vi "TDMS File Merge.vi"(0 "serial input channel":string="SI0", 5 "tdms file directory":path, 7 "progress ref":refnum<vi>, 11 "error in":errorcluster) -> (15 "error out":errorcluster)   [LabVIEW 2023, in "GettingStarted_Common_148X_Host.lvlib"]
uses:
  GettingStarted_Common_148X_Host.lvlib
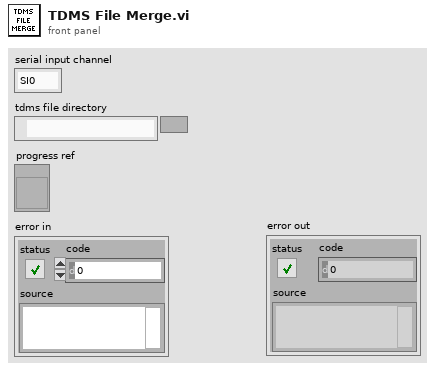
[diagram p1: front panel]
types:
  T1 = enum16{"open", "open or create", "create or replace", "create", "open (read-only)"}
  T2 = enum16{"big-endian, network order", "native, host order", "little-endian"}
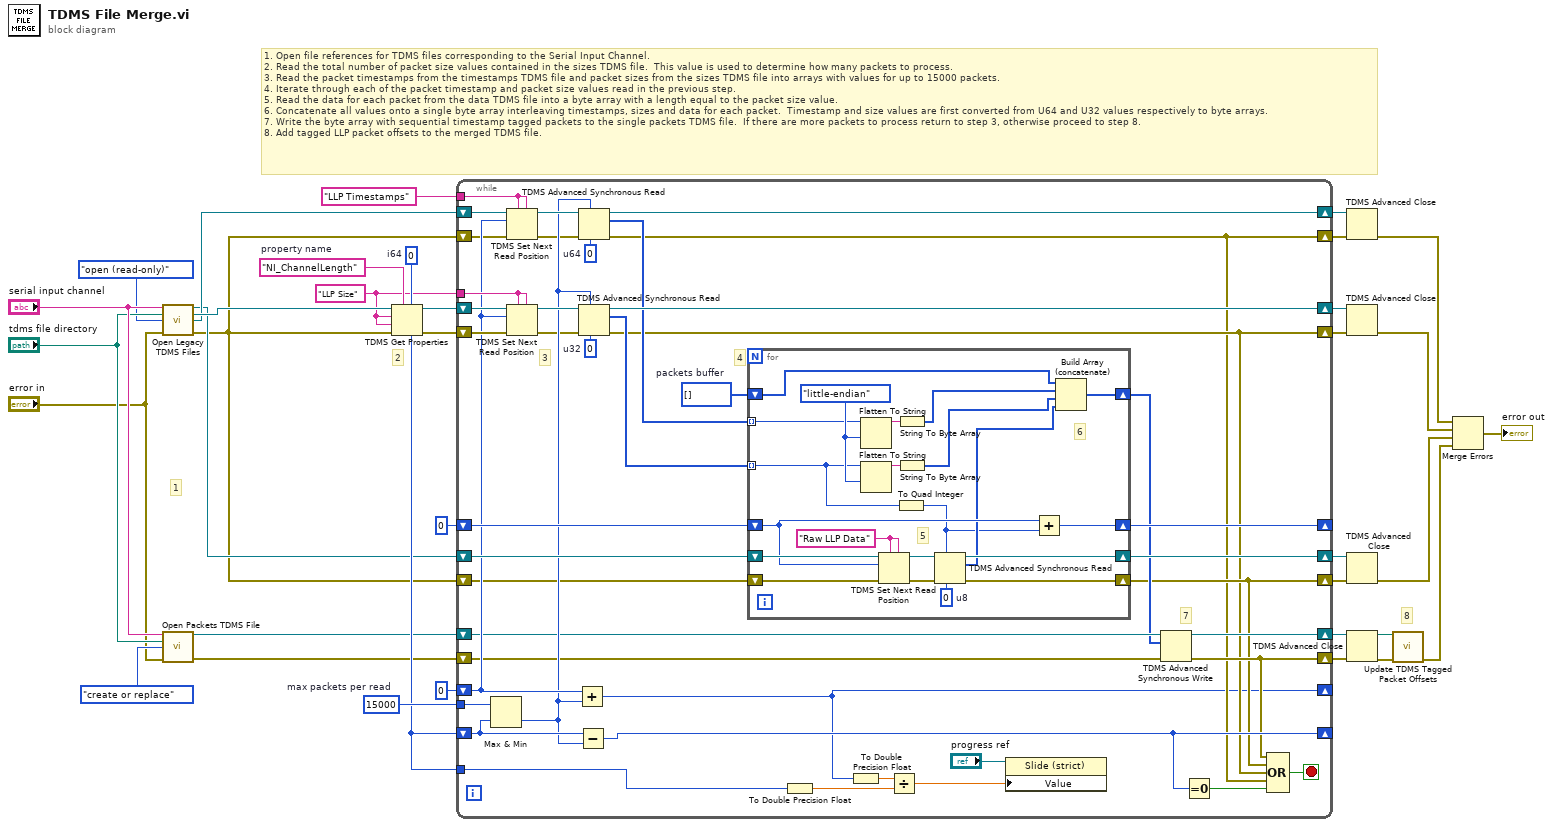
[diagram p0: block diagram]
diagram:
  w33 = i64 15000  # max packets per read
  w16 = "LLP Size" ("channel and group name")
  w35 = i64 0  # i64
  w36 = "NI_ChannelLength"  # property name
  # "2"
  # "8"
  # "1"
  # "1. Open file references for TDMS files corresponding to the Serial Input Channel.\n2. Read the total number of packet size values contained in the sizes TDMS file.  This value is used to determine how many packets to process.\n3. Read the packet timestamps from the timestamps TDMS file and packet sizes from the sizes TDMS file into arrays with values for up to 15000 packets.\n4. Iterate through each of the packet timestamp and packet size values read in the previous step.\n5. Read the data for each packet from the data TDMS file into a byte array with a length equal to the packet size value.\n6. Concatenate all values onto a single byte array interleaving timestamps, sizes and data for each packet.  Timestamp and size values are first converted from U64 and U32 values respectively to byte arrays.\n7. Write the byte array with sequential timestamp tagged packets to the single packets TDMS file.  If there are more packets to process return to step 3, otherwise proceed to step 8.\n8. Add tagged LLP packet offsets to the merged TDMS file."
  n1 = call "Open Legacy TDMS Files.vi"("serial input channel"="serial input channel", "base tdms file path"="tdms file directory", "file operation type"=T1."open (read-only)", "error in (no error)"="error in") -> ("data file ref"=w28:refnum<k34>, "sizes file ref"=w30:refnum<k34>, "timestamp file ref"=w29:refnum<k34>, "error out"=w15:errorcluster)  [unwired: 8 in]
  n2 = call "Open Packets TDMS File.vi"("serial input channel"="serial input channel", "base tdms file path"="tdms file directory", "file operation type"=T1."create or replace", "error in"="error in") -> ("packets file ref"=w23:refnum<k34>, "error out"=w14:errorcluster)  [unwired: 10 in]
  n3 = TDMS Get Properties(5:w35, 7:w36, 8:w15, 9:w16, 10:w16, 11:w30) -> (0:w34:errorcluster, 3:w31:refnum<k34>, 4:w32:i64)  [unwired: 3 out]
  n4 = while {
    shift-right: [w70] -> w17
    shift-left: w29 -> [w73]
    shift-right: [w45] -> w22
    shift-left: w34 -> [w77]
    shift-right: [w53] -> _
    shift-left: w32 -> [w78]
    tunnel: w33 -> [w79]
    tunnel: w32 -> [w39]
    shift-right: [w74] -> w18
    shift-left: w31 -> [w72]
    tunnel: w16 -> [w65]
    shift-right: [w40] -> _
    shift-left: i64 0 -> [w60]
    shift-right: [w63] -> w20
    shift-left: w28 -> [w66]
    shift-right: [w61] -> _
    shift-left: i64 0 ("initial file offset") -> [w64]
    shift-right: [w56] -> w19
    shift-left: w23 -> [w58]
    shift-right: [w46] -> w12
    shift-left: w15 -> [w51]
    shift-right: [w44] -> w13
    shift-left: w15 -> [w52]
    shift-right: [w47] -> w11
    shift-left: w14 -> [w50]
    tunnel: "LLP Timestamps" ("channel and group name") -> [w49]
    stop <- w43 stop-if-true
    w62 = u8[] []  # packets buffer
    w69 = u64 0  # u64
    w75 = u32 0  # u32
    # "4"
    # "7"
    # "3"
    n5 = Max & Min(x=w79, y=w78) -> (min(x,y)=w59:i64)  [unwired: 1 out]
    n6 = TDMS Set Next Read Position(5:w49, 7:w49, 8:w52, 10:w60, 11:w73) -> (0:w54:errorcluster, 3:w71:refnum<k34>)  [unwired: 1 in]
    n7 = TDMS Set Next Read Position(5:w65, 7:w65, 8:w77, 10:w60, 11:w72) -> (0:w55:errorcluster, 3:w76:refnum<k34>)  [unwired: 1 in]
    n8 = Add(x=w60, y=w59) -> (x+y=w40:i64)
    n9 = Subtract(x=w78, y=w59) -> (x-y=w53:i64)
    n10 = TDMS Advanced Synchronous Read(6:w69, 7:w59, 8:w54, 11:w71) -> (0:w44:errorcluster, 2:w67:u64[], 3:w70:refnum<k34>)  [unwired: 1 out]
    n11 = TDMS Advanced Synchronous Read(6:w75, 7:w59, 8:w55, 11:w76) -> (0:w45:errorcluster, 2:w68:u32[], 3:w74:refnum<k34>)  [unwired: 1 out]
    n12 = for {
      tunnel: w68 -> [w81] mode=indexing
      tunnel: w67 -> [w82] mode=indexing
      shift-right: [w93] -> w61
      shift-left: w64 -> [w94]
      shift-right: [w98] -> w46
      shift-left: w51 -> [w88]
      shift-right: [w96] -> w63
      shift-left: w66 -> [w100]
      shift-right: [w90] -> w57
      shift-left: w62 -> [w91]
      w83 = T2."little-endian" ("byte order (0:big-endian, network order)")
      w89 = "Raw LLP Data" ("channel and group name")
      w95 = u8 0  # u8
      # "6"
      # "5"
      n13 = Flatten To String(anything=w82, byte order (0:big-endian, network order)=w83) -> (data string=w85:string)  [unwired: 2 in, 2 out]
      n14 = Flatten To String(anything=w81, byte order (0:big-endian, network order)=w83) -> (data string=w87:string)  [unwired: 2 in, 2 out]
      n15 = TDMS Set Next Read Position(5:w89, 7:w89, 8:w88, 10:w94, 11:w100) -> (0:w99:errorcluster, 3:w97:refnum<k34>)  [unwired: 1 in]
      n16 = To Quad Integer(1:w81) -> (0:w80:i64)
      n17 = String To Byte Array(string=w85) -> (unsigned byte array=w84:u8[])
      n18 = String To Byte Array(string=w87) -> (unsigned byte array=w86:u8[])
      n19 = TDMS Advanced Synchronous Read(6:w95, 7:w80, 8:w99, 11:w97) -> (0:w98:errorcluster, 2:w92:u8[], 3:w96:refnum<k34>)  [unwired: 1 out]
      n20 = Add(x=w94, y=w80) -> (x+y=w93:i64)
      n21 = Build Array (concatenate)(w91, w84, w86, w92) -> (w90:u8[])
    }
    n22 = To Double Precision Float(number=w39) -> (double precision float=w41:dbl)
    n23 = To Double Precision Float(number=w40) -> (double precision float=w42:dbl)
    n24 = Divide(x=w42, y=w41) -> (x/y=w37:dbl)
    n25 = property class="Slide (strict)"(reference="progress ref", "Value"=w37) -> ()  [unwired: 1 in, 2 out]
    n26 = TDMS Advanced Synchronous Write(8:w50, 10:w57, 11:w58) -> (0:w47:errorcluster, 3:w56:refnum<k34>)
    n27 = Equal To 0?(x=w53) -> (x = 0?=w48:bool)
    n28 = Compound Arithmetic op=OR(w47, w46, w45, w44, w48) -> (w43:bool)
  }
  n29 = TDMS Advanced Close(8:w13, 11:w17) -> (0:w8:errorcluster)  [unwired: 2 in, 1 out]
  n30 = TDMS Advanced Close(8:w22, 11:w18) -> (0:w7:errorcluster)  [unwired: 2 in, 1 out]
  n31 = TDMS Advanced Close(8:w12, 11:w20) -> (0:w6:errorcluster)  [unwired: 2 in, 1 out]
  n32 = TDMS Advanced Close(8:w11, 11:w19) -> (0:w2:errorcluster, 3:w3:path)  [unwired: 2 in]
  n33 = call "Update TDMS Tagged Packet Offsets.vi"("llp tagged packet file path"=w3, "error in"=w2) -> ("error out"=w1:errorcluster)  [unwired: 12 in, 1 out]
  n34 = Merge Errors(w8, w7, w6, w1) -> (→"error out":errorcluster)
